vi "test Send Stop.vi"(8 "error in (no error)":errorcluster, 11 "TestCase in":refnum<class "Test TCP Nested Endpoint Nonforwarded Messages.lvclass">) -> (0 "error out":errorcluster, 3 "TestCase out":refnum<class "Test TCP Nested Endpoint Nonforwarded Messages.lvclass">)   [LabVIEW 2020, in "Test TCP Nested Endpoint Nonforwarded Messages.lvclass"]
uses:
  Test TCP Nested Endpoint Nonforwarded Messages.lvclass
  <vilib>/addons/_JKI Toolkits/VI Tester/TestCase.llb/TestCase.lvclass
  <vilib>/ActorFramework/Message Queue/Message Queue.lvclass
  <vilib>/ActorFramework/Message Dequeuer/Message Dequeuer.lvclass
  <vilib>/ActorFramework/LastAck/Last Ack.lvclass
  <vilib>/ActorFramework/Stop Msg/Stop Msg.lvclass
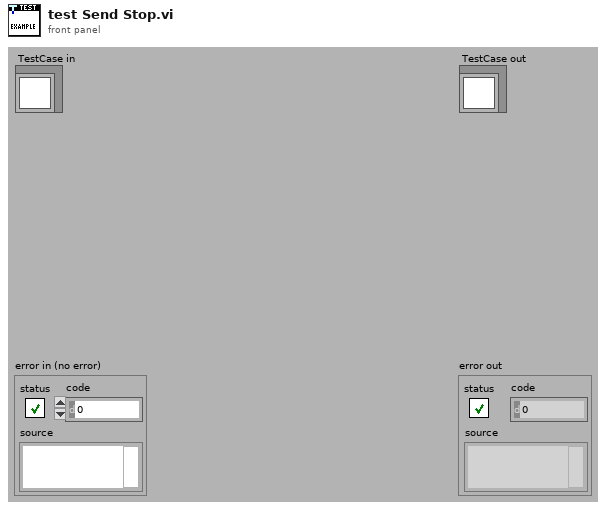
[diagram p1: front panel]
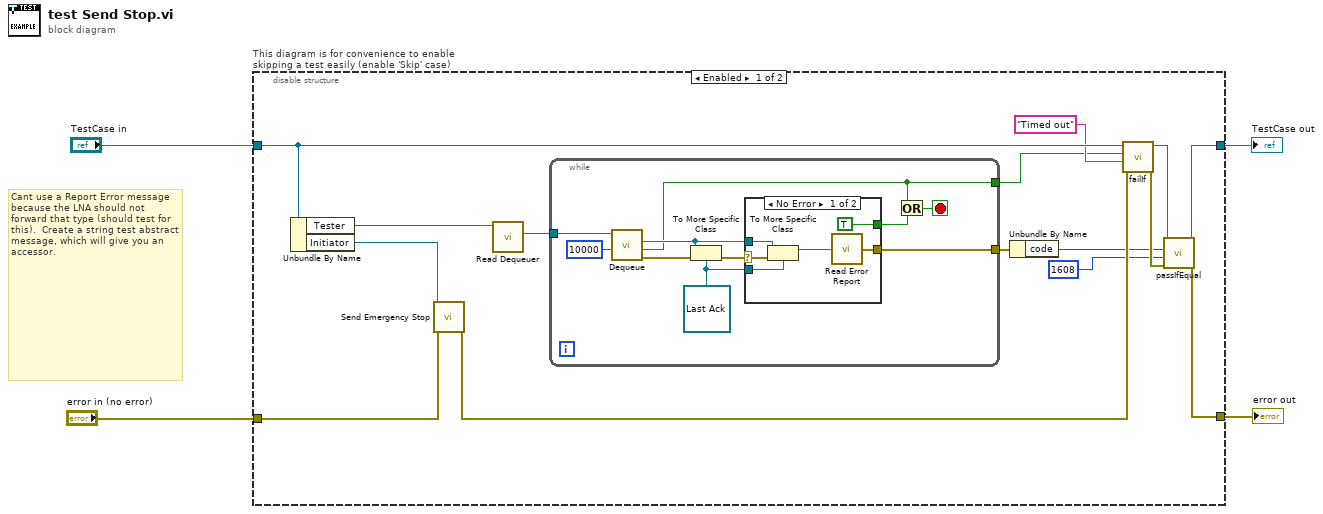
[diagram p0: block diagram]
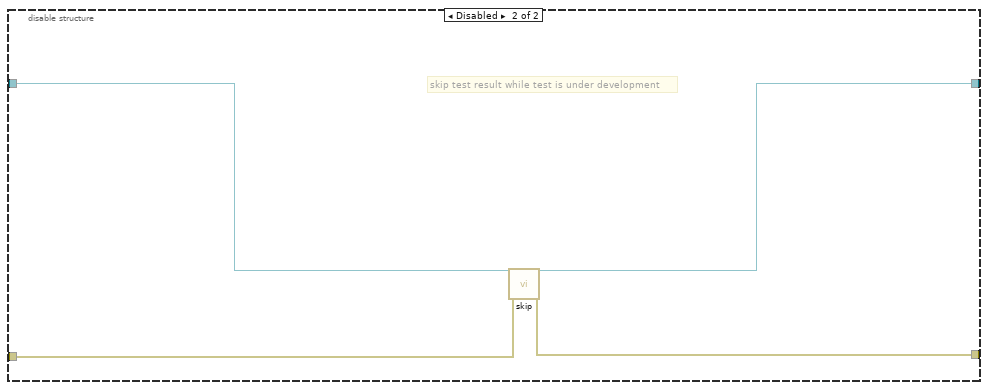
[diagram p3: hidden frame]
diagram:
  # "Cant use a Report Error message because the LNA should not forward that type (should test for this).  Create a string test abstract message, which will give you an accessor."
  n1 = disable-structure "This diagram is for convenience to enable skipping a test easily (enable 'Skip' case)" shown="Enabled" {
    disable-tunnel: "TestCase in" -> [w15 w39]
    disable-tunnel: [w19 w37] -> w1
    disable-tunnel: [w18 w38] -> w3
    disable-tunnel: "error in (no error)" -> [w9 w36]
    frame Enabled {
      n2 = Unbundle By Name(w15) -> ("Tester"=w16:refnum<class "Message Queue.lvclass">, "Initiator"=w7:refnum<class "Message Enqueuer.lvclass">)
      n3 = call <vilib>:"Send Emergency Stop.vi"("error in (no error)"=w9, "Message Enqueuer"=w7) -> ("error out"=w8:errorcluster)  [unwired: 9 in]
      n4 = call <vilib>:"Read Dequeuer.vi"("Message Queue"=w16) -> ("Message Dequeuer"=w17:refnum<class "Message Dequeuer.lvclass">)  [unwired: 10 in]
      n5 = while {
        tunnel: w17 -> [w29]
        tunnel: [w22] -> w10
        tunnel: [w23] -> w11
        stop <- w20 stop-if-true
        w24 = refnum<class "Last Ack.lvclass"> refnum ("Last Ack")
        n6 = call <vilib>:"Dequeue.vi"("timeout in ms (-1)"=10000, "Message Dequeuer in"=w29) -> ("error out"=w27:errorcluster, "timed out?"=w23:bool, "Message"=w25:refnum<class "Message.lvclass">)  [unwired: 5 in, 2 out]
        n7 = To More Specific Class(target class=w24, reference=w25, error in=w27) -> (error out=w26:errorcluster)  [unwired: 1 out]
        n8 = case shown="No Error" w26 {
          selector: w26 -> [w35 _]
          tunnel: w25 -> [w34 _]
          tunnel: w24 -> [w33 _]
          tunnel: [w31 _] -> w22
          tunnel: [TRUE _] -> w21
          frame No Error {
            n9 = To More Specific Class(target class=w33, reference=w34, error in=w35) -> (specific class reference=w32:refnum<class "Last Ack.lvclass">)  [unwired: 1 out]
            n10 = call <vilib>:"Read Error Report.vi"("Last Ack"=w32) -> ("error report"=w31:errorcluster)
          }
          frame Error {
          }
        }
        n11 = Or(x=w23, y=w21) -> (x .or. y?=w20:bool)
      }
      n12 = Unbundle By Name(w10) -> ("code"=w6:i32)
      n13 = call-dynamic "failIf.vi"("error in (no error)"=w8, "message (\"\")"="Timed out" ("message (\"\")"), "fail"=w11, "TestCase in"=w15) -> ("error out"=w13:errorcluster, "TestCase out"=w14:refnum<class "Test TCP Nested Endpoint Nonforwarded Messages.lvclass">)  [unwired: 6 in]
      n14 = call-dynamic "passIfEqual.vi"("error in (no error)"=w13, "y"=1608 ("code"), "x"=w6, "TestCase in"=w14) -> ("error out"=w18:errorcluster, "TestCase out"=w19:refnum<class "Test TCP Nested Endpoint Nonforwarded Messages.lvclass">)  [unwired: 6 in]
    }
    frame Disabled {
      # "skip test result while test is under development"
      n15 = call <vilib>:"skip.vi"("error in (no error)"=w36, "TestCase in"=w39) -> ("error out"=w38:errorcluster, "TestCase out"=w37:refnum<class "Test TCP Nested Endpoint Nonforwarded Messages.lvclass">)  [unwired: 8 in]
    }
  }
  "error out" <- w3
  "TestCase out" <- w1
